vi "Alphabetize Case-Sensitive Cluster Constant Target.vi"() -> ()   [LabVIEW 2018, in "Tests.lvlib" / "Toolkit.lvlib"]
uses:
  Toolkit.lvlib
panel:
  out "Boolean":bool
  in  "String":string
  in  "Numeric":dbl
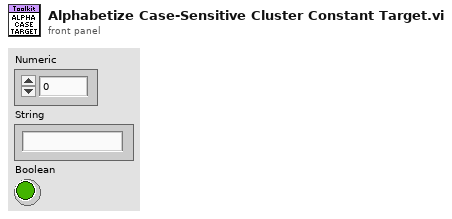
[diagram p1: front panel]
types:
  T1 = cluster{"string4":string, "sTring3":string, "STring2":string, "String1":string}
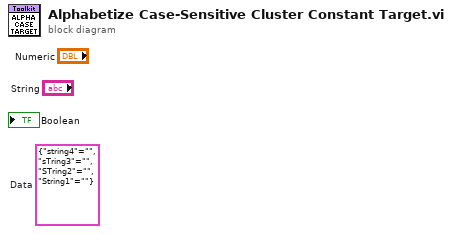
[diagram p0: block diagram]
diagram:
  (unwired) T1 {"string4"="", "sTring3"="", "STring2"="", "String1"=""}  # Data
